vi "Set DO IONames.vi"(8 "error in (no error)":errorcluster, 10 "DO IONames":string[](array[string]), 11 "DAQ in":refnum<class "DAQ.lvclass">) -> (0 "error out":errorcluster, 3 "DAQ out":refnum<class "DAQ.lvclass">)   [LabVIEW 2017, in "DAQ.lvclass"]
doc: "Developed by Kevin Thompson\nkevin@thompsonengineering.net\n\nCopyright 2018-2020\nThompson Engineering, LLC"
uses:
  DAQ.lvclass
  DAQ.lvclass/DAQ.ctl
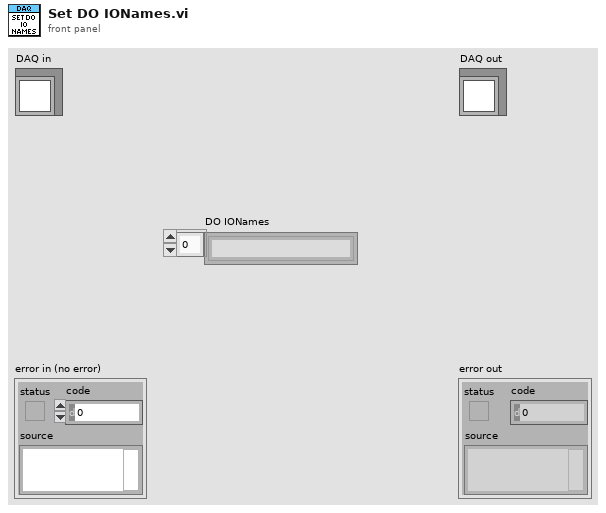
[diagram p1: front panel]
types:
  T1 = typedef "DAQ.lvclass/TD Obj Data_DAQ--cluster.ctl" = cluster{"DAQ&TDMS State Data":T2, "DAQ Settings":T4, "DI TaskNames":string[], "AI TaskNames":string[], "DI IONames":string[], "DI SchemNames":string[], "DO IONames":string[], "DO SchemNames":string[], "AI IONames":string[], "AI SchemNames":string[], "AO IONames":string[], "AO SchemNames":string[]}
  T2 = typedef "DAQ.lvclass/TD DAQ&TDMS State Data--cluster.ctl" = cluster{"DAQState":T3, "vData":variant}
  T3 = typedef "DAQ.lvclass/TD DaqState--enum.ctl" = enum16{"Unknown", "Stopped", "Running", "Error"}
  T4 = typedef "DAQ.lvclass/TD DAQ Settings--cluster.ctl" = cluster{"Simulate DAQ":bool, "DI Settings":T5[], "AI Settings":T6[], "Relay IONames":string[], "AO IONames":string[], "AO NChan SingleTask":bool}
  T5 = typedef "DAQ.lvclass/TD DI Instrument Settings--cluster.ctl" = cluster{"Disable":bool, "DI TaskName":string, "DI RefreshIntv":i32}
  T6 = typedef "DAQ.lvclass/TD AI Instrument Settings--cluster.ctl" = cluster{"Disable":bool, "AI TaskName":string, "AI InstSettings":T7, "SimAI Ranges":T8}
  T7 = typedef "DAQ.lvclass/TD AI InstSettings--cluster.ctl" = cluster{"DaqRate":dbl, "NumSamples":i32}
  T8 = typedef "DAQ.lvclass/TD SimAI Ranges--cluster.ctl" = cluster{"lo":dbl, "hi":dbl}
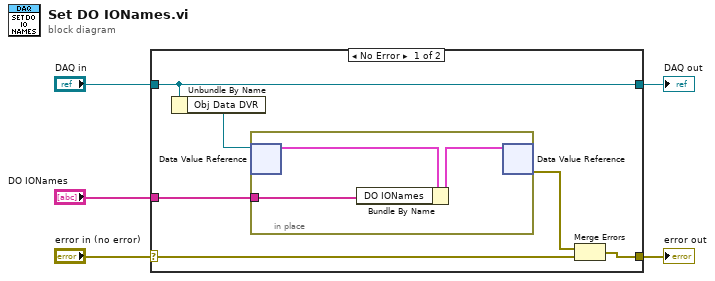
[diagram p0: block diagram]
diagram:
  n1 = case shown="No Error" "error in (no error)" {
    selector: "error in (no error)" -> [w11 w15]
    tunnel: [w9 w15] -> w4
    tunnel: [w10 w16] -> w2
    tunnel: "DAQ in" -> [w10 w16]
    tunnel: "DO IONames" -> [w7 _]
    frame No Error {
      n2 = Unbundle By Name(w10) -> ("Obj Data DVR"=w8:refnum<data-value>)
      n3 = in-place {
        in-place-border: w7 -> [w12]
        n4 = in-place-dvr #1(w8) -> (w14:T1)  [unwired: 1 out]
        n5 = Bundle By Name(cluster=w14, "DO IONames"=w12) -> (w13:T1)
        n6 = in-place-dvr #1(w13) -> (w6:errorcluster)  [unwired: 1 out]
      }
      n7 = Merge Errors(w6, w11) -> (w9:errorcluster)
    }
    frame Error {
    }
  }
  "error out" <- w4
  "DAQ out" <- w2
